vi "Update Zone Indicators.vi"(8 "error in":errorcluster, 9 "Step":i32, 10 "Elapsed Time":dbl, 11 "Zone Setup Array":cluster{"Zone Selector":string, "Timing":dbl}[](array[cluster])) -> (0 "error out":errorcluster, 3 "Zone Indicators":T1)   [LabVIEW 2020]
doc: "This VI updates the Zone indicators."
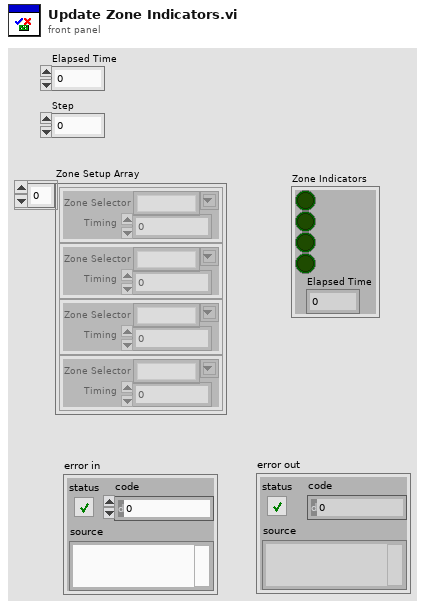
[diagram p1: front panel]
types:
  T1 = cluster{bool, bool, bool, bool, "Elapsed Time":dbl}
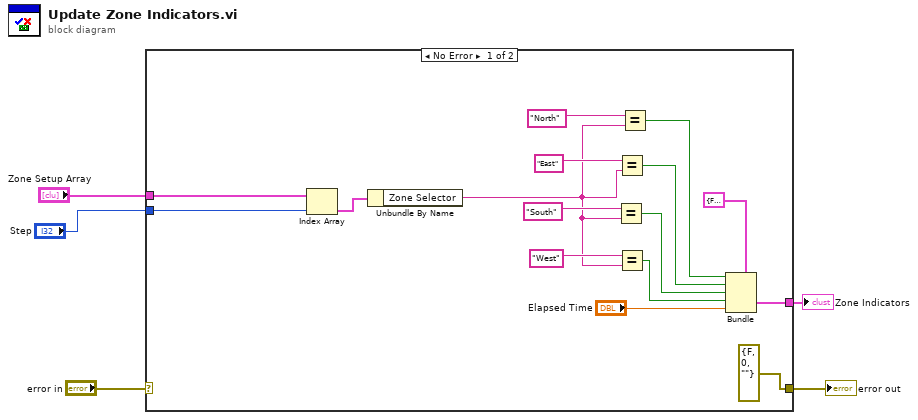
[diagram p0: block diagram]
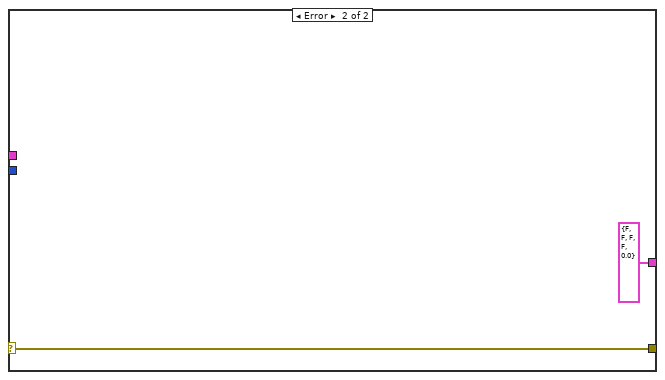
[diagram p2: hidden frame]
diagram:
  n1 = case shown="No Error" "error in" {
    selector: "error in" -> [_ w23]
    tunnel: [errorcluster {"status"=FALSE, "code"=0, "source"=""} ("error IO") w23] -> w4
    tunnel: [w9 T1 {FALSE, FALSE, FALSE, FALSE, "Elapsed Time"=0.0} ("cluster")] -> w3
    tunnel: "Zone Setup Array" -> [w7 _]
    tunnel: "Step" -> [w6 _]
    frame No Error {
      n2 = Index Array(array=w7, index=w6) -> (element=w21:cluster{"Zone Selector":string, "Timing":dbl})
      n3 = Unbundle By Name(w21) -> ("Zone Selector"=w14:string)
      n4 = Equal?(x="South" ("Zone Selector"), y=w14) -> (x = y?=w11:bool)
      n5 = Equal?(x="East" ("Zone Selector"), y=w14) -> (x = y?=w12:bool)
      n6 = Equal?(x="West" ("Zone Selector"), y=w14) -> (x = y?=w10:bool)
      n7 = Equal?(x="North" ("Zone Selector"), y=w14) -> (x = y?=w13:bool)
      n8 = Bundle(cluster=T1 {FALSE, FALSE, FALSE, FALSE, "Elapsed Time"=0.0}, w13, w12, w11, w10, "Elapsed Time"="Elapsed Time") -> (w9:T1)
    }
    frame Error {
    }
  }
  "error out" <- w4
  "Zone Indicators" <- w3
